vi "Script Non-Dynamic Square Run Output.vi"(11 "Project":refnum<vi>) -> (0 "error out":errorcluster)   [LabVIEW 2020]
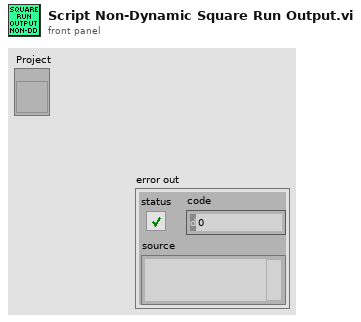
[diagram p1: front panel]
types:
  T1 = enum16{"Invalid Wire Rule", "Required", "Recommended", "Optional", "Dynamic Dispatch"}
  T2 = enum16{"Invalid Wire Rule", "Required", "Recommended", "Optional", "Dynamic Dispatch"}[]
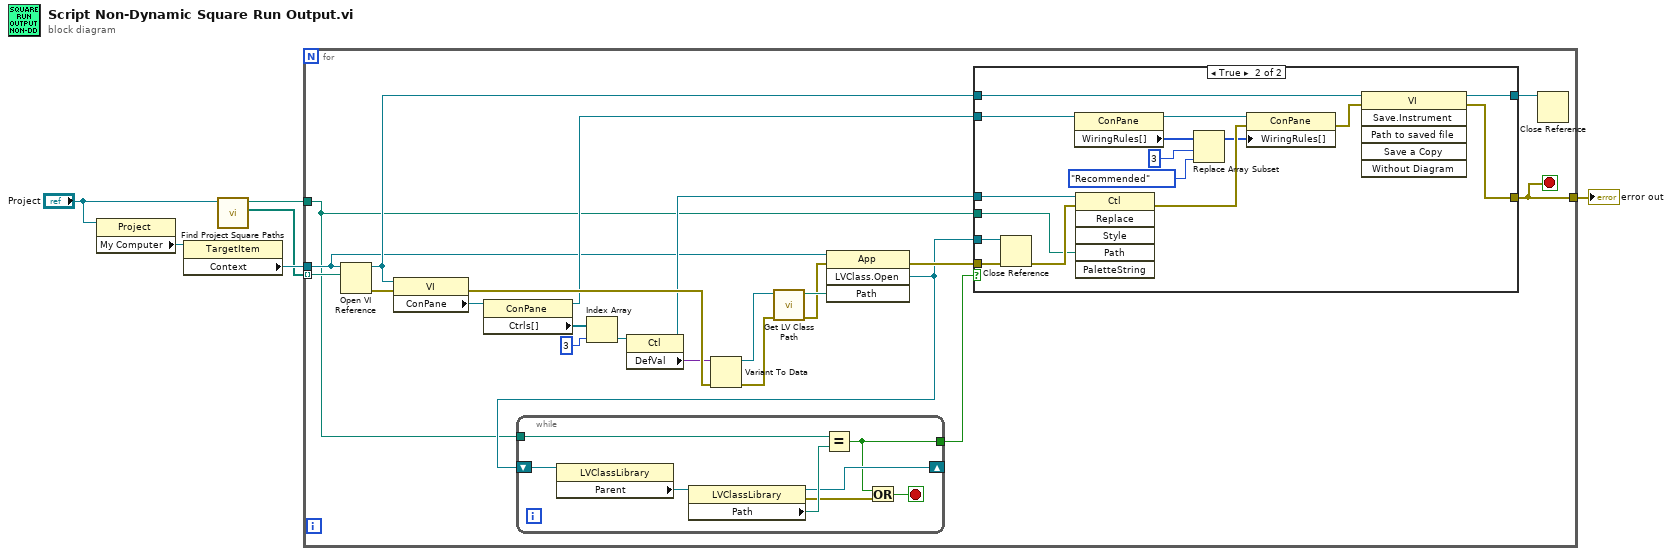
[diagram p0: block diagram]
diagram:
  n1 = property class="Project"(reference="Project") -> ("My Computer"=w4:refnum<vi>)  [unwired: 1 in, 2 out]
  n2 = property class="TargetItem"(reference=w4) -> ("Context"=w3:refnum<vi>)  [unwired: 1 in, 2 out]
  n3 = call "Find Project Square Paths.vi"("Project"="Project") -> ("Square Run VIs"=w2:path[], "Base Square"=w6:path)  [unwired: 8 in, 1 out]
  n4 = for {
    tunnel: w6 -> [w7]
    tunnel: w2 -> [w10] mode=indexing
    tunnel: w3 -> [w11]
    tunnel: [w8] -> w1
    stop <- w8 stop-if-true
    n5 = Open VI Reference(application reference (local)=w11, vi path=w10) -> (vi reference=w13:refnum<vi>, error out=w26:errorcluster)  [unwired: 4 in]
    n6 = property class="VI"(reference=w13, error in=w26) -> (error out=w27:errorcluster, "ConPane"=w25:refnum<vi>)  [unwired: 1 out]
    n7 = property class="ConPane"(reference=w25) -> (reference out=w14:refnum<vi>, "Ctrls[]"=w24:refnum<vi>[])  [unwired: 1 in, 1 out]
    n8 = Index Array(array=w24, index=3) -> (element=w22:refnum<vi>)
    n9 = property class="Ctl"(reference=w22) -> (reference out=w16:refnum<vi>, "DefVal"=w21:variant)  [unwired: 1 in, 1 out]
    n10 = Variant To Data(error in=w27, Variant=w21) -> (data=w20:refnum<class>, error out=w28:errorcluster)  [unwired: 1 in]
    n11 = call <vilib>:"Get LV Class Path.vi"("error in (no error)"=w28, "object"=w20) -> ("error out"=w18:errorcluster, "class path"=w19:path)  [unwired: 8 in]
    n12 = invoke class="App" method="LVClass.Open"(reference=w11, error in=w18, "Path"=w19) -> (error out=w15:errorcluster, "LVClass.Open"=w9:refnum<vi>)  [unwired: 1 in, 2 out]
    n13 = while {
      shift-right: [w31] -> _
      shift-left: w9 -> [w36]
      tunnel: [w30] -> w17
      tunnel: w7 -> [w29]
      stop <- w33 stop-if-true
      n14 = property class="LVClassLibrary"(reference=w36) -> ("Parent"=w35:refnum<vi>)  [unwired: 1 in, 2 out]
      n15 = property class="LVClassLibrary"(reference=w35) -> (reference out=w31:refnum<vi>, error out=w32:errorcluster, "Path"=w34:path)  [unwired: 1 in]
      n16 = Equal?(x=w29, y=w34) -> (x = y?=w30:bool)
      n17 = Or(x=w30, y=w32) -> (x .or. y?=w33:bool)
    }
    n18 = case shown="True" w17 {
      tunnel: w16 -> [_ w54]
      tunnel: w15 -> [w38 w53]
      tunnel: [w38 w42] -> w8
      tunnel: w14 -> [_ w51]
      tunnel: w13 -> [w37 w44]
      tunnel: [w37 w41] -> w12
      tunnel: w9 -> [_ w40]
      tunnel: w7 -> [_ w39]
      frame False {
      }
      frame True {
        n19 = Close Reference(reference=w40, error in (no error)=w53) -> (error out=w52:errorcluster)
        n20 = property class="ConPane"(reference=w51) -> (reference out=w47:refnum<vi>, "WiringRules[]"=w50:T2)  [unwired: 1 in, 1 out]
        n21 = invoke class="Ctl" method="Replace"(reference=w54, error in=w52, "Path"=w39) -> (error out=w46:errorcluster)  [unwired: 3 in, 5 out]
        n22 = Replace Array Subset(array=w50, new element=T1."Recommended" ("new element/subarray"), index=3) -> (w45:T2)
        n23 = property class="ConPane"(reference=w47, error in=w46, "WiringRules[]"=w45) -> (error out=w43:errorcluster)  [unwired: 1 out]
        n24 = invoke class="VI" method="Save.Instrument"(reference=w44, error in=w43) -> (reference out=w41:refnum<vi>, error out=w42:errorcluster)  [unwired: 4 in, 4 out]
      }
    }
    n25 = Close Reference(reference=w12) -> ()  [unwired: 1 in, 1 out]
  }
  "error out" <- w1
